vi "Draw Boat Trace.vi"(4 "Radius (px)":dbl=5.0, 6 "circle color":u32(colorbox)=16777215, 9 "Position":cluster{"X":i32, "Y":i32}, 11 "Image In":T1) -> (3 "Image Out":T1)   [LabVIEW 2013]
doc: "Places a dot on the map showing where the boat has been.\n\n4/5/2014\nMac-I Crowell"
uses:
  <vilib>/vision/Image Controls.llb/IMAQ Image.ctl
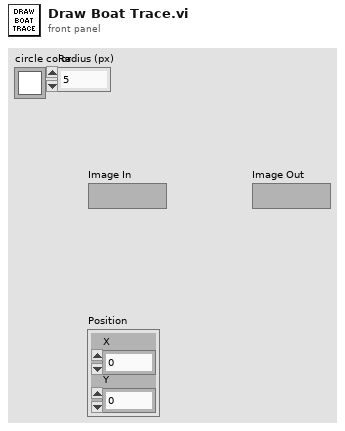
[diagram p1: front panel]
types:
  T1 = typedef "IMAQ Image.ctl" = refnum<image>
  T2 = cluster{"Left":i32, "Top":i32, "Right":i32, "Bottom":i32}
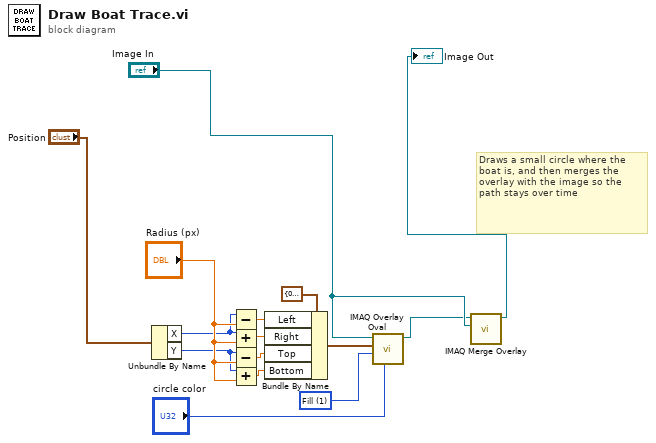
[diagram p0: block diagram]
diagram:
  w6 = u32 1 items=["Frame", "Fill"] ("Drawing Mode (Frame)")
  # "Draws a small circle where the boat is, and then merges the overlay with the image so the path stays over time"
  n1 = Unbundle By Name("Position") -> ("X"=w12:i32, "Y"=w13:i32)
  n2 = Subtract(x=w12, y="Radius (px)") -> (x-y=w9:dbl)
  n3 = Add(x=w12, y="Radius (px)") -> (x+y=w8:dbl)
  n4 = Subtract(x=w13, y="Radius (px)") -> (x-y=w11:dbl)
  n5 = Add(x=w13, y="Radius (px)") -> (x+y=w10:dbl)
  n6 = Bundle By Name(cluster=T2 {"Left"=0, "Top"=0, "Right"=0, "Bottom"=0} ("Bounding Rectangle"), "Left"=w9, "Right"=w8, "Top"=w11, "Bottom"=w10) -> (w15:T2)
  n7 = call "IMAQ Overlay Oval"("Color"="circle color", "Drawing Mode (Frame)"=w6, "Bounding Rectangle"=w15, "Image"="Image In") -> ("Image Out"=w2:T1)  [unwired: 6 in, 1 out]
  n8 = call "IMAQ Merge Overlay"("Image Dst"="Image In", "Image Src"=w2) -> ("Image Dst Out"=→"Image Out":T1)  [unwired: 8 in, 1 out]
